vi "速度报文计算公式.vi"(1 "速度":dbl(slide) scale=-30.0..30.0) -> (0 "输出角速度报文":string)   [LabVIEW 2023]
panel:
  in  "选项卡控件":enum32{"选项卡 1", "选项卡 2"}(tab)
  out "角速度16进制报文":string
  out "十进制数":i32
  out "二进制":string
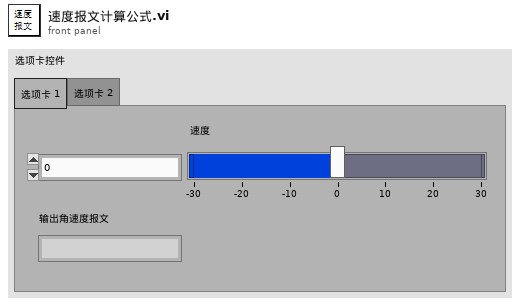
[diagram p1: front panel]
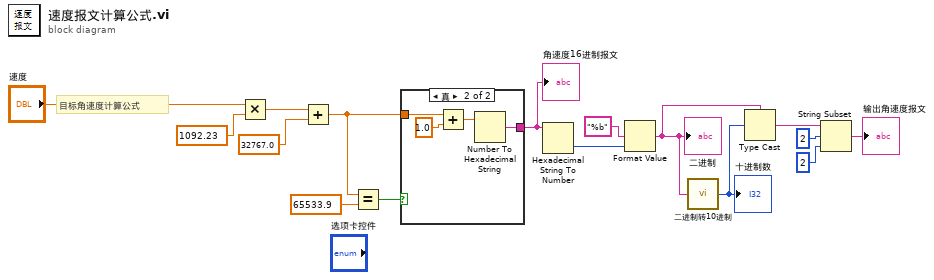
[diagram p0: block diagram]
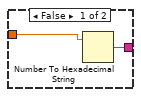
[diagram p2: hidden frame]
diagram:
  # "目标角速度计算公式"
  n1 = Multiply(x="速度", y=1092.23) -> (x*y=w15:dbl)
  n2 = Add(x=w15, y=32767.0) -> (x+y=w7:dbl)
  n3 = Equal?(x=w7, y=65533.9) -> (x = y?=w1:bool)
  n4 = case shown="真" w1 {
    tunnel: w7 -> [w18 w21]
    tunnel: [w17 w22] -> w6
    frame False {
      n5 = Number To Hexadecimal String(2:w18) -> (0:w17:string)  [unwired: 1 in]
    }
    frame True {
      n6 = Add(x=w21, y=1.0) -> (x+y=w19:dbl)
      n7 = Number To Hexadecimal String(2:w19) -> (0:w22:string)  [unwired: 1 in]
    }
  }
  "角速度16进制报文" <- w6
  n8 = Hexadecimal String To Number(string=w6) -> (number=w10:u32)  [unwired: 2 in, 1 out]
  n9 = Format Value(format string="%b" ("格式字符串"), value (0)=w10) -> (output string=w8:string)  [unwired: 1 in]
  "二进制" <- w8
  n10 = call "二进制转10进制.vi"("字符串"=w8) -> ("十进制数"=w9:i32)
  "十进制数" <- w9
  n11 = Type Cast(type=w8, x=w9) -> (*(type *) &x=w5:string)
  n12 = String Subset(string=w5, offset (0)=2 ("偏移量(0)"), length (rest)=2 ("长度（剩余）")) -> (substring=→"输出角速度报文":string)
